vi "update_menus.vi"(7 "UpdateMenuCommand":T1, 8 "error in (no error)":errorcluster) -> (0 "error out":errorcluster, 2 "Right Menu":T3, 3 "Left Menu":T2)   [LabVIEW 2017]
uses:
  controls/Left Menu.ctl
  controls/Right Menu.ctl
  controls/UpdateMenuCmd.ctl
  controls/Menu.ctl
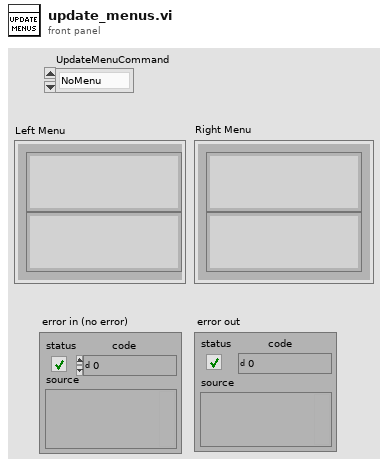
[diagram p1: front panel]
types:
  T1 = typedef "UpdateMenuCmd.ctl" = enum16{"NoMenu", "MainMenu"}
  T2 = typedef "Right Menu.ctl" = cluster{"Indicator1":string, "Indicator4":string}
  T3 = typedef "Left Menu.ctl" = cluster{"Indicator1":string, "Indicator4":string}
  T4 = typedef "Menu.ctl" = cluster{string, "Menu 0":string}
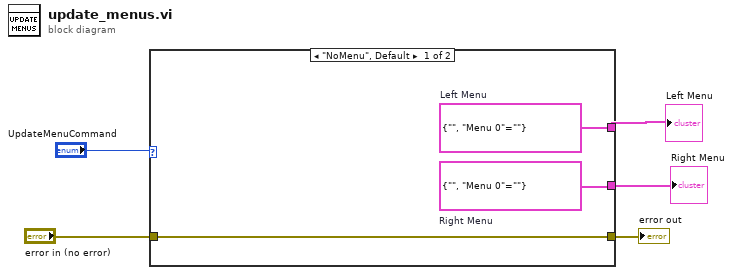
[diagram p0: block diagram]
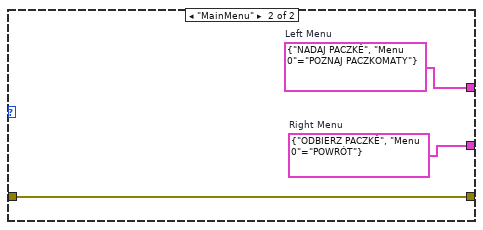
[diagram p2: hidden frame]
diagram:
  n1 = case shown="\"NoMenu\", Default" "UpdateMenuCommand" {
    tunnel: "error in (no error)" -> [w6 w11]
    tunnel: [w6 w11] -> w4
    tunnel: [w8 w10] -> w2
    tunnel: [w7 w9] -> w1
    frame "NoMenu", Default {
      w7 = T4 {"", "Menu 0"=""}  # Right Menu
      w8 = T4 {"", "Menu 0"=""}  # Left Menu
    }
    frame "MainMenu" {
      w9 = T4 {"ODBIERZ PACZKÊ", "Menu 0"="POWRÓT"}  # Right Menu
      w10 = T4 {"NADAJ PACZKÊ", "Menu 0"="POZNAJ PACZKOMATY"}  # Left Menu
    }
  }
  "Right Menu" <- w1
  "Left Menu" <- w2
  "error out" <- w4
